vi "Set Value Change Trigger.vi"(7 "Trigger Direction":T2, 8 "error in (no error)":errorcluster, 10 "Value Change Trigger":T1, 11 "Item Ref in":T3 format="%.0x") -> (0 "error out":errorcluster, 3 "Item Ref out":T3 format="%.0x")   [LabVIEW 2015, in "Waveform Data Logger Shared.lvlib"]
uses:
  Waveform Data Logger Shared.lvlib
  <vilib>/NI Veristand/Custom Device API/Custom Device Item Ref.ctl
  Types/Trigger Direction.ctl
  Types/Value Change Trigger.ctl
  Globals/Property Strings.vi
  <vilib>/NI Veristand/Custom Device API/Set Item Property (Double).vi
  <vilib>/NI VeriStand/Custom Device API/Custom Device API.lvlib
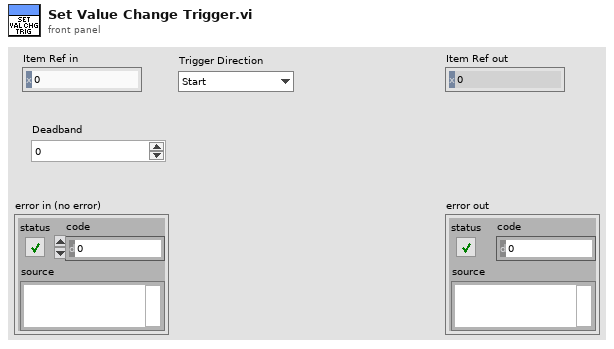
[diagram p1: front panel]
types:
  T1 = typedef "Waveform Data Logger Shared.lvlib/Value Change Trigger.ctl" = cluster{"Deadband":dbl}
  T2 = typedef "Waveform Data Logger Shared.lvlib/Trigger Direction.ctl" = enum16{"Start", "Stop"}
  T3 = typedef "Custom Device API.lvlib/Custom Device Item Ref.ctl" = u64
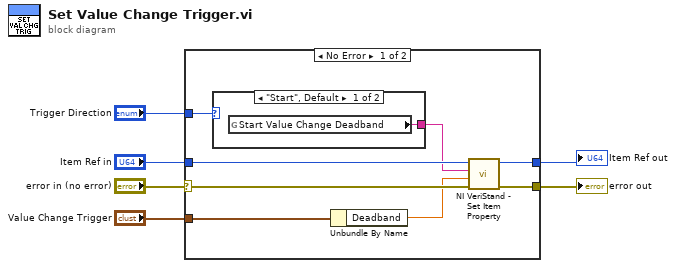
[diagram p0: block diagram]
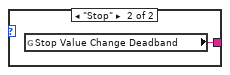
[diagram p2: hidden frame]
diagram:
  n1 = case shown="No Error" "error in (no error)" {
    selector: "error in (no error)" -> [w12 w17]
    tunnel: [w8 w18] -> w6
    tunnel: [w7 w17] -> w5
    tunnel: "Item Ref in" -> [w14 w18]
    tunnel: "Value Change Trigger" -> [w13 _]
    tunnel: "Trigger Direction" -> [w11 _]
    frame No Error {
      n2 = case shown="\"Start\", Default" w11 {
        tunnel: [w15 w16] -> w9
        frame "Start", Default {
          n3 = global read "Property Strings.vi" "Start Value Change Deadband"() -> (w15:string)
        }
        frame "Stop" {
          n4 = global read "Property Strings.vi" "Stop Value Change Deadband"() -> (w16:string)
        }
      }
      n5 = Unbundle By Name(w13) -> ("Deadband"=w10:dbl)
      n6 = call-poly <vilib>:"NI VeriStand - Set Item Property.vi"("error in (no error)"=w12, "Value"=w10, "Property Name"=w9, "Item Ref in"=w14) -> ("error out"=w7:errorcluster, "Item Ref out"=w8:T3)  [unwired: 5 in, 1 out]
    }
    frame Error {
    }
  }
  "Item Ref out" <- w6
  "error out" <- w5
